vi "Read From Connection.vi"(8 "error in (no error)":errorcluster, 9 "Timeout (ms)":i32, 10 "Bytes to Read":i32, 11 "ProtectedConnectionReader in":refnum<class "ProtectedConnectionReader.lvclass">) -> (0 "error out":errorcluster, 2 "TimeOut?":bool, 3 "Data":string)   [LabVIEW 2019, in "ProtectedConnectionReader.lvclass"]
uses:
  <vilib>/gpm_packages/@cs/Network-interface/Source/ProtectedConnectionReader/ProtectedConnectionReader.lvclass
  <vilib>/gpm_packages/@cs/Network-interface/Source/ProtectedConnectionReader/ProtectedConnectionReader.lvclass/ProtectedConnectionReader.ctl
  <vilib>/gpm_packages/@cs/Network-interface/Source/Connection Reference/Connection Reference/Connection Reference.lvclass/Connection Reference.ctl
  <vilib>/gpm_packages/@cs/Network-interface/Source/Connection Reference/IConnection/IConnection.lvclass
  <vilib>/gpm_packages/@cs/Network-interface/Source/Connection Reference/Connection Reference/Connection Reference.lvclass
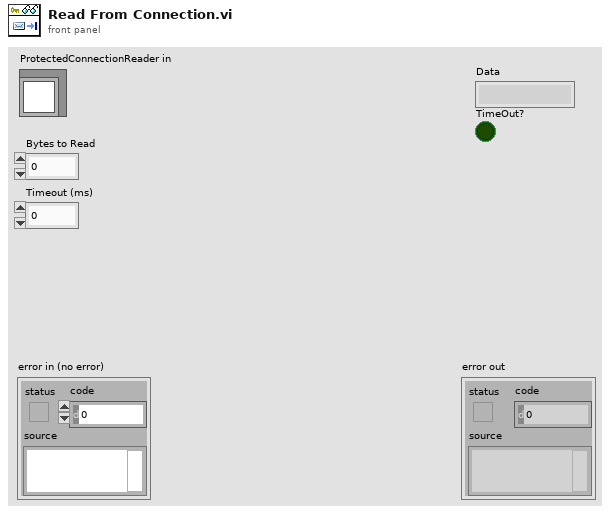
[diagram p1: front panel]
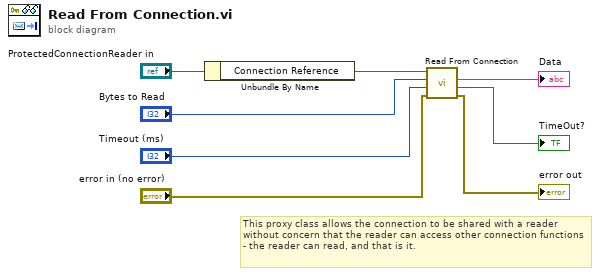
[diagram p0: block diagram]
diagram:
  # "This proxy class allows the connection to be shared with a reader without concern that the reader can access other connection functions - the reader can read, and that is it."
  n1 = Unbundle By Name("ProtectedConnectionReader in") -> ("Connection Reference"=w7:refnum<data-value>)
  n2 = call <vilib>:"Read From Connection.vi"("error in (no error)"="error in (no error)", "Timeout (ms)"="Timeout (ms)", "Bytes to Read"="Bytes to Read", "Connection Reference In"=w7) -> ("error out"=→"error out":errorcluster, "TimeOut?"=→"TimeOut?":bool, "Data"=→"Data":string)  [unwired: 4 in, 1 out]
